vi "Validate Credentials Local Machine.vi"(8 "error in (no error)":errorcluster, 10 "password":string, 11 "userName":string) -> (0 "error out":errorcluster, 3 "valid":bool)   [LabVIEW 2017, in "Windows Security.lvlib"]
doc: "Validate the credentials against the domain."
uses:
  Windows Security.lvlib
  System.DirectoryServices.AccountManagement
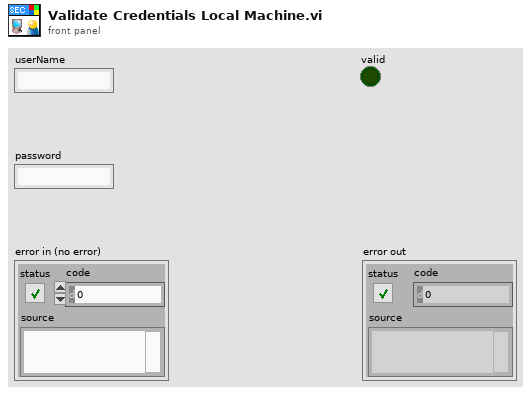
[diagram p1: front panel]
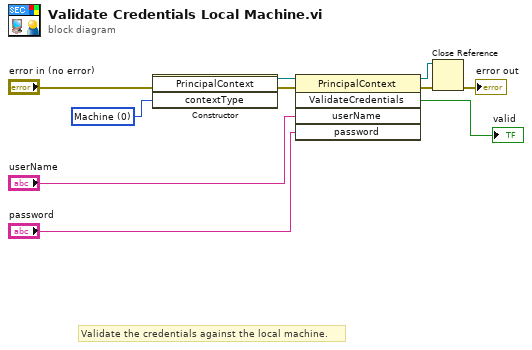
[diagram p0: block diagram]
diagram:
  w10 = 0 items=["Machine", "Domain", "ApplicationDirectory"] ("contextType")
  # "Validate the credentials against the local machine."
  n1 = constructor class="PrincipalContext"(error in="error in (no error)", "contextType"=w10) -> (reference out=w8:refnum<k24>, error out=w7:errorcluster)  [unwired: 2 in, 2 out]
  n2 = invoke class="PrincipalContext" method="ValidateCredentials"(reference=w8, error in=w7, "userName"="userName", "password"="password") -> (reference out=w5:refnum<k24>, error out=w6:errorcluster, "ValidateCredentials"=→"valid":bool)  [unwired: 1 in, 2 out]
  n3 = Close Reference(reference=w5, error in (no error)=w6) -> (error out=→"error out":errorcluster)
